vi "Set laser power.vi"(10 "Laser Power":dbl(slide) min=0.0 max=120.0 step=1.0 scale=0.0..100.0 scale format="%.1f", 11 "VISA resource name":refnum<visa-resource-name>) -> (3 "VISA resource name out":refnum<visa-resource-name>)   [LabVIEW 2017]
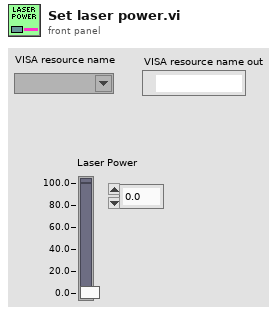
[diagram p1: front panel]
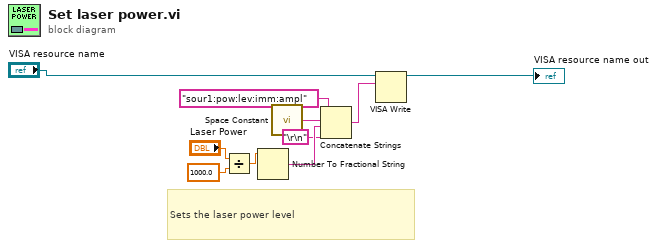
[diagram p0: block diagram]
diagram:
  # "Sets the laser power level"
  n1 = Divide(x="Laser Power", y=1000.0) -> (x/y=w5:dbl)
  n2 = Number To Fractional String(number=w5) -> (F-format string=w8:string)  [unwired: 3 in]
  n3 = call <vilib>:"Space Constant.vi"() -> ("String"=w9:string)
  n4 = Concatenate Strings("sour1:pow:lev:imm:ampl", w9, w8, "\r\n") -> (w4:string)
  n5 = VISA Write(VISA resource name="VISA resource name", write buffer=w4) -> (VISA resource name out=→"VISA resource name out":refnum<visa-resource-name>)  [unwired: 1 in, 2 out]
